vi "Get Touched.vi"(8 "error in (no error)":errorcluster, 11 "TermLine in":refnum<class "TermLine.lvclass">) -> (0 "error out":errorcluster, 2 "Touched":bool, 3 "TermLine out":refnum<class "TermLine.lvclass">)   [LabVIEW 2020, in "Terminal.lvlib" / "TermLine.lvclass"]
uses:
  TermLine.lvclass
  TermLine.lvclass/TermLine.ctl
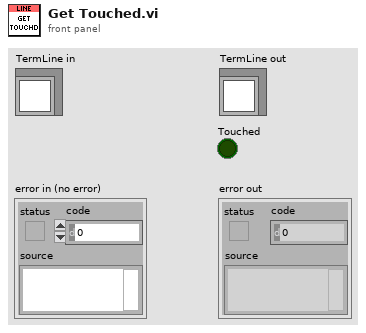
[diagram p1: front panel]
types:
  T1 = typedef "Terminal.lvlib/TermLine.lvclass/Ref Data.ctl" = cluster{"Chars":T2[], "Width":i32, "Touched":bool}
  T2 = typedef "Terminal.lvlib/Term Char.ctl" = cluster{"Char":string, "Attributes":T3}
  T3 = typedef "Terminal.lvlib/Text Attributes.ctl" = cluster{"FG":u32, "BG":u32, "Bold":bool, "Italic":bool, "Underline":bool, "Strike":bool, "Inverse":bool}
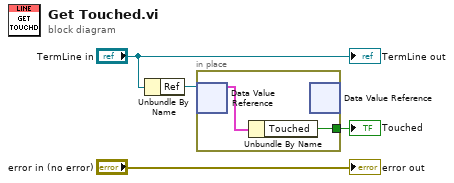
[diagram p0: block diagram]
diagram:
  n1 = Unbundle By Name("TermLine in") -> ("Ref"=w3:refnum<data-value>)
  n2 = in-place {
    in-place-border: [w5] -> w1
    n3 = in-place-dvr #1(w3) -> (w6:T1)  [unwired: 1 out]
    n4 = Unbundle By Name(w6) -> ("Touched"=w5:bool)
    n5 = in-place-dvr #1() -> ()  [unwired: 1 in, 2 out]
  }
  "Touched" <- w1
  "error out" <- "error in (no error)"
  "TermLine out" <- "TermLine in"
